vi "Set Channel Status.vi"(8 "Status Info":T2, 9 "Data Type":string, 10 "My System Status":T1(ring), 11 "Real Data":sgl[](array[numeric])) -> (3 "Channel Statuses":u32[](array[numeric]))   [LabVIEW 2013, in "Customer.TestSLATE.Mnemonic.lvlib"]
uses:
  Customer.TestSLATE.Mnemonic.lvlib
  <vilib>/Test SLATE/CONTROLS/ChannelStatusBit.ctl
  <vilib>/Test SLATE/Test SLATE.lvlib
panel:
  # "Channel Status Alarm Bit Values\n       1 - Saturated\n       2 - Conversion Error\n       4 - In Calibration\n       8 - In Diagnostics Mode\n     16 - Bad Coded\n     32 - NaN"
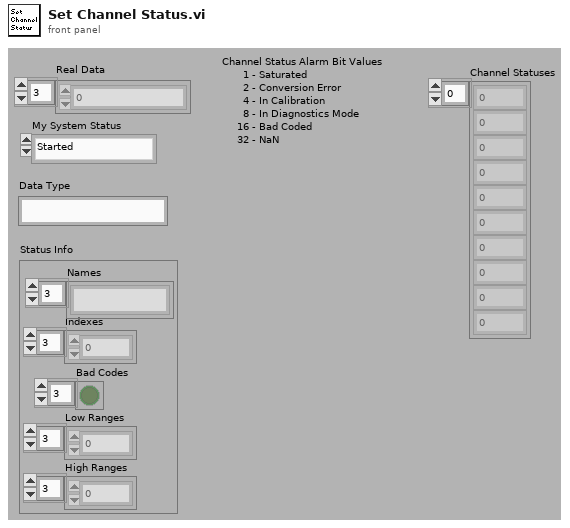
[diagram p1: front panel]
types:
  T1 = enum16{"Started", "Stopped", "Initializing", "Acquiring", "Calibrating", "Diagnostics", "Inactive"}
  T2 = cluster{"Indexes":i32[], "Names":string[], "Bad Codes":bool[], "Low Ranges":sgl[], "High Ranges":sgl[]}
  T3 = typedef "Test SLATE.lvlib/ChannelStatusBit.ctl" = enum32{"Saturated", "Conversion Error", "in Calibration", "in Diagnostics", "Bad Coded", "NaN"}
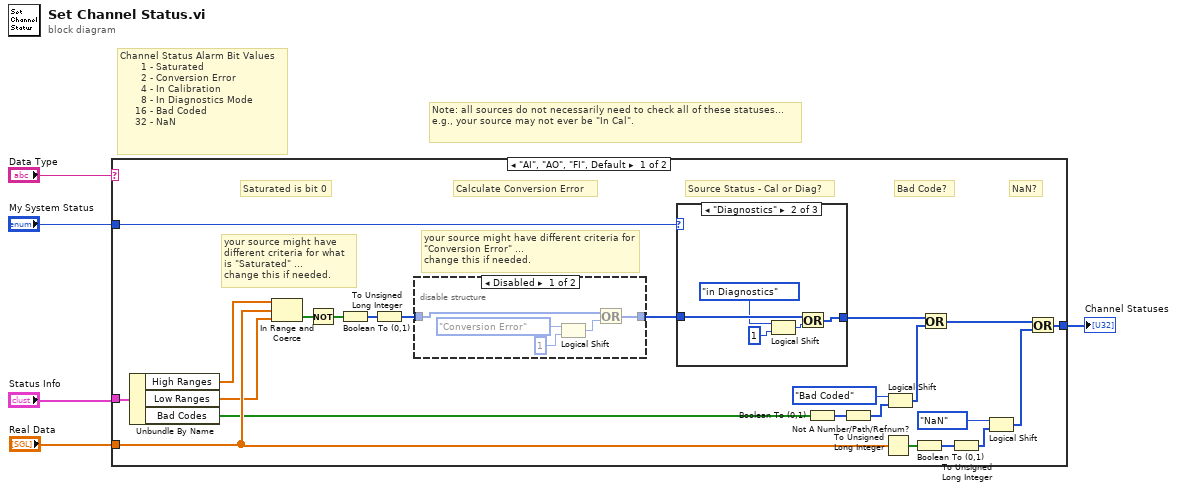
[diagram p0: block diagram]
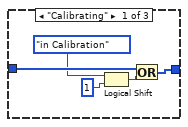
[diagram p2: hidden frame]
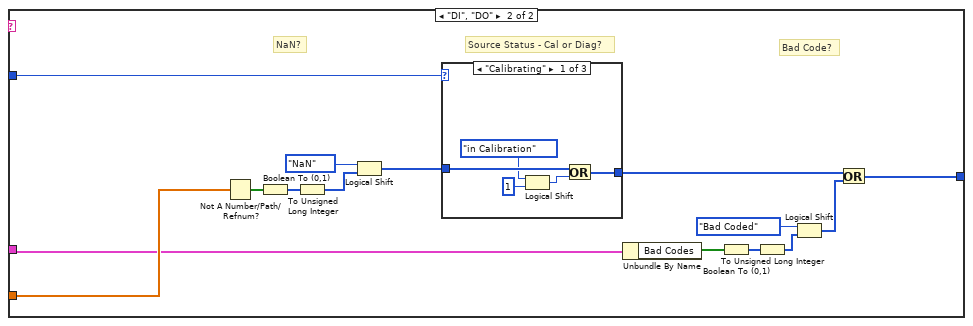
[diagram p5: hidden frame]
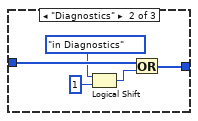
[diagram p6: hidden frame]
diagram:
  # "Note: all sources do not necessarily need to check all of these statuses...\ne.g., your source may not ever be \"In Cal\"."
  # "Channel Status Alarm Bit Values\n       1 - Saturated\n       2 - Conversion Error\n       4 - In Calibration\n       8 - In Diagnostics Mode\n     16 - Bad Coded\n     32 - NaN"
  n1 = case shown="\"AI\", \"AO\", \"FI\", Default" "Data Type" {
    tunnel: [w13 w46] -> w1
    tunnel: "Real Data" -> [w11 w51]
    tunnel: "Status Info" -> [w10 w50]
    tunnel: "My System Status" -> [w6 w48]
    frame "AI", "AO", "FI", Default {
      # "NaN?"
      # "your source might have different criteria for \"Conversion Error\" ...\nchange this if needed."
      # "your source might have \ndifferent criteria for what \nis \"Saturated\" ...\nchange this if needed."
      # "Bad Code?"
      # "Source Status - Cal or Diag?"
      # "Calculate Conversion Error"
      # "Saturated is bit 0"
      n2 = Unbundle By Name(w10) -> ("High Ranges"=w9:sgl[], "Low Ranges"=w8:sgl[], "Bad Codes"=w7:bool[])
      n3 = In Range and Coerce(upper limit=w9, x=w11, lower limit=w8) -> (In Range?=w28:bool[])  [unwired: 1 out]
      n4 = Not(x=w28) -> (.not. x?=w12:bool[])
      n5 = Boolean To (0,1)(Boolean=w12) -> (0, 1=w27:i16[])
      n6 = To Unsigned Long Integer(number=w27) -> (unsigned 32bit integer=w26:u32[])
      n7 = disable-structure shown="Disabled" {
        disable-tunnel: w26 -> [w44 w45]
        disable-tunnel: [w41 w45] -> w25
        frame Disabled {
          n8 = Logical Shift(y=ChannelStatusBit."Conversion Error" ("Channel Status Bit"), x=u32 1) -> (x << y=w43:u32)
          n9 = Or(x=w44, y=w43) -> (x .or. y?=w41:u32[])
        }
        frame Enabled {
        }
      }
      n10 = case shown="\"Diagnostics\"" w6 {
        tunnel: w25 -> [w33 w38 w39]
        tunnel: [w29 w34 w39] -> w22
        frame "Calibrating" {
          n11 = Logical Shift(y=ChannelStatusBit."in Calibration" ("Channel Status Bit"), x=u32 1) -> (x << y=w32:u32)
          n12 = Or(x=w33, y=w32) -> (x .or. y?=w29:u32[])
        }
        frame "Diagnostics" {
          n13 = Logical Shift(y=ChannelStatusBit."in Diagnostics" ("Channel Status Bit"), x=u32 1) -> (x << y=w37:u32)
          n14 = Or(x=w38, y=w37) -> (x .or. y?=w34:u32[])
        }
        frame "Inactive", Default {
        }
      }
      n15 = Boolean To (0,1)(Boolean=w7) -> (0, 1=w21:i16[])
      n16 = To Unsigned Long Integer(number=w21) -> (unsigned 32bit integer=w20:u32[])
      n17 = Not A Number/Path/Refnum?(number/path/refnum=w11) -> (NaN/Path/Refnum?=w15:bool[])
      n18 = Logical Shift(y=ChannelStatusBit."Bad Coded" ("Channel Status Bit"), x=w20) -> (x << y=w23:u32[])
      n19 = Boolean To (0,1)(Boolean=w15) -> (0, 1=w14:i16[])
      n20 = Or(x=w22, y=w23) -> (x .or. y?=w16:u32[])
      n21 = To Unsigned Long Integer(number=w14) -> (unsigned 32bit integer=w19:u32[])
      n22 = Logical Shift(y=ChannelStatusBit."NaN" ("Channel Status Bit"), x=w19) -> (x << y=w18:u32[])
      n23 = Or(x=w16, y=w18) -> (x .or. y?=w13:u32[])
    }
    frame "DI", "DO" {
      # "NaN?"
      # "Bad Code?"
      # "Source Status - Cal or Diag?"
      n24 = Not A Number/Path/Refnum?(number/path/refnum=w51) -> (NaN/Path/Refnum?=w53:bool[])
      n25 = Boolean To (0,1)(Boolean=w53) -> (0, 1=w52:i16[])
      n26 = To Unsigned Long Integer(number=w52) -> (unsigned 32bit integer=w55:u32[])
      n27 = Logical Shift(y=ChannelStatusBit."NaN" ("Channel Status Bit"), x=w55) -> (x << y=w47:u32[])
      n28 = case shown="\"Calibrating\"" w48 {
        tunnel: w47 -> [w65 w70 w71]
        tunnel: [w61 w66 w71] -> w58
        frame "Calibrating" {
          n29 = Logical Shift(y=ChannelStatusBit."in Calibration" ("Channel Status Bit"), x=u32 1) -> (x << y=w64:u32)
          n30 = Or(x=w65, y=w64) -> (x .or. y?=w61:u32[])
        }
        frame "Diagnostics" {
          n31 = Logical Shift(y=ChannelStatusBit."in Diagnostics" ("Channel Status Bit"), x=u32 1) -> (x << y=w69:u32)
          n32 = Or(x=w70, y=w69) -> (x .or. y?=w66:u32[])
        }
        frame "Inactive", Default {
        }
      }
      n33 = Unbundle By Name(w50) -> ("Bad Codes"=w49:bool[])
      n34 = Boolean To (0,1)(Boolean=w49) -> (0, 1=w57:i16[])
      n35 = To Unsigned Long Integer(number=w57) -> (unsigned 32bit integer=w56:u32[])
      n36 = Logical Shift(y=ChannelStatusBit."Bad Coded" ("Channel Status Bit"), x=w56) -> (x << y=w59:u32[])
      n37 = Or(x=w58, y=w59) -> (x .or. y?=w46:u32[])
    }
  }
  "Channel Statuses" <- w1
